vi "gascell.vi"() -> ()   [LabVIEW 2014, in "Panels.lvlib"]
uses:
  Panels.lvlib
  CSlibraries-extern/DimLVEvent/DimIndicators/DimIndicators.lvlib
  CSlibraries/UtilityLib/UtilityLib.lvlib
  CSCore/CSSystem/CoreLib/CoreLib.lvlib
  CSlibraries/UtilityLib/UtilityLib.valueStatus.ctl
  CSlibraries-extern/DimLVEvent/LVDimInterface/LVDimInterface.lvlib
  Instance           1 15Saved   gascell .vi
  CSCore/CSSystem/CoreLib/CoreLib.string 2 byte array.vi
  CSCore/CSSystem/CoreLib/CoreLib.double 2 byte array.vi
  CSCore/CSSystem/CoreLib/CoreLib.short 2 byte array.vi
  CSlibraries-extern/DimLVEvent/DimIndicators/DimIndicators.numericType.ctl
  CSCore/BaseProcess/BaseProcess.descriptor string definition.ctl
  CSCore/BaseProcess/BaseProcess.lvlib
  CSCore/CSSystem/CoreDefs/CoreDefs.rawDataType.ctl
  CSCore/CSSystem/CoreDefs/CoreDefs.call_type.ctl
  CSlibraries-extern/DimLVEvent/DimIndicators/DimIndicators.numericArrayType.ctl
  CSlibraries-extern/DimLVEvent/DimIndicators/DimIndicators.anyType.ctl
panel:
  in  "ListOfBases_Data":T1={"data"="NOLINK", "no link"=TRUE, "quality"=-1, "timeStamp"=0.0}
  in  "SetFileLocation_Data":T1={"data"="NOLINK", "no link"=TRUE, "quality"=-1, "timeStamp"=0.0}
  in  "GasCellBase_SetValueInfoData":T2={"data"=[0.0, 400.0, 2.0], "no link"=FALSE, "quality"=0, "timeStamp"=3265902002.226}
  in  "Flower2":bool
  in  "Flower3":bool
  in  "NozzlePlate":bool
  in  "NozzleVolt":bool
  in  "Flower1":bool
  in  "Flower4":bool
  in  "Ring21":bool
  in  "Ring18":bool
  in  "Ring17":bool
  in  "Ring3":bool
  in  "Ring1":bool
  in  "GasCellPIR_MonData":T3={"data"=inf, "no link"=FALSE, "quality"=1, "timeStamp"=3265902002.211}
  in  "N4PumpPIR_MonData":T3={"data"=inf, "no link"=FALSE, "quality"=1, "timeStamp"=3265902002.211}
  out "GasCellPIR_Mon":dbl=inf format="%.4f"
  out "N4PumpPIR_Mon":dbl=inf format="%.4f"
  in  "NozzlePlate_SetValueInfoData":T2={"data"=[0.0, 400.0, 2.0], "no link"=FALSE, "quality"=0, "timeStamp"=3265902002.226}
  in  "GasCellBase_SetData":T2={"data"=[0.0, 0.0, 0.0, 0.0], "no link"=FALSE, "quality"=0, "timeStamp"=3265902003.554}
  in  "NozzleVolt_SetValueInfoData":T2={"data"=[-120.0, 120.0, 2.0], "no link"=FALSE, "quality"=0, "timeStamp"=3265902002.226}
  in  "NozzlePlate_SetData":T2={"data"=[0.0, 0.0, 0.0, 0.0], "no link"=FALSE, "quality"=0, "timeStamp"=3265902003.57}
  in  "NozzlePlate_MonData":T3={"data"=inf, "no link"=FALSE, "quality"=1, "timeStamp"=3265902002.195}
  out "Ring3_Mon":dbl=inf format="%.4f"
  out "Ring1_Mon":dbl=inf format="%.4f"
  out "i ref out":refnum<vi>
  in  "Last Loaded File_Data":T1
  out "FileUpToDate":bool=TRUE caption="Parameter Changed"
  in  "Close All Panels":bool
  in  "Ring3_SetValueInfoData":T2={"data"=[0.0, 2989.8, 2.0], "no link"=FALSE, "quality"=0, "timeStamp"=3265902002.211}
  in  "Ring17_SetValueInfoData":T2={"data"=[0.0, 2988.4, 2.0], "no link"=FALSE, "quality"=0, "timeStamp"=3265902002.226}
  in  "Ring18_SetValueInfoData":T2={"data"=[0.0, 2984.0, 2.0], "no link"=FALSE, "quality"=0, "timeStamp"=3265902002.226}
  in  "Ring21_SetValueInfoData":T2={"data"=[0.0, 1488.3, 2.0], "no link"=FALSE, "quality"=0, "timeStamp"=3265902002.226}
  in  "Flower1_SetValueInfoData":T2={"data"=[0.0, 1487.9, 2.0], "no link"=FALSE, "quality"=0, "timeStamp"=3265902002.226}
  in  "Flower2_SetValueInfoData":T2={"data"=[0.0, 1486.0, 2.0], "no link"=FALSE, "quality"=0, "timeStamp"=3265902002.226}
  in  "Flower3_SetValueInfoData":T2={"data"=[0.0, 1488.7, 2.0], "no link"=FALSE, "quality"=0, "timeStamp"=3265902002.226}
  in  "Flower4_SetValueInfoData":T2={"data"=[0.0, 500.0, -1.0], "no link"=FALSE, "quality"=0, "timeStamp"=3265902002.226}
  in  "Ring1_SetValueInfoData":T2={"data"=[0.0, 2997.3, 2.0], "no link"=FALSE, "quality"=0, "timeStamp"=3265902002.211}
  in  "Ring1_SetData":T2={"data"=[0.0, 0.0, 0.0, 0.0], "no link"=FALSE, "quality"=0, "timeStamp"=3265902003.554}
  in  "Flower4_SetData":T2={"data"=[0.0, 0.0, 0.0, 0.0], "no link"=FALSE, "quality"=0, "timeStamp"=3265902003.539}
  in  "Flower3_SetData":T2={"data"=[0.0, 0.0, 0.0, 0.0], "no link"=FALSE, "quality"=0, "timeStamp"=3265902003.57}
  in  "Flower2_SetData":T2={"data"=[0.0, 0.0, 0.0, 0.0], "no link"=FALSE, "quality"=0, "timeStamp"=3265902003.554}
  in  "Flower1_SetData":T2={"data"=[0.0, 0.0, 0.0, 0.0], "no link"=FALSE, "quality"=0, "timeStamp"=3265902003.554}
  in  "Ring21_SetData":T2={"data"=[0.0, 0.0, 0.0, 0.0], "no link"=FALSE, "quality"=0, "timeStamp"=3265902003.554}
  in  "Ring18_SetData":T2={"data"=[0.0, 0.0, 0.0, 0.0], "no link"=FALSE, "quality"=0, "timeStamp"=3265902003.554}
  in  "Ring17_SetData":T2={"data"=[0.0, 0.0, 0.0, 0.0], "no link"=FALSE, "quality"=0, "timeStamp"=3265902003.554}
  in  "Ring3_SetData":T2={"data"=[0.0, 0.0, 0.0, 0.0], "no link"=FALSE, "quality"=0, "timeStamp"=3265902003.554}
  in  "NozzleVolt_SetData":T2={"data"=[0.0, 0.0, 0.0, 0.0], "no link"=FALSE, "quality"=0, "timeStamp"=3265902003.57}
  in  "call cluster in":T4={"Object"="", "Selector"="", "CallType"=enum."synchronous", "Async Object"="", "Async Selector"="", "Data Descriptor"="", "Data"=[], "Error #"=0, "Expire"=0}
  in  "GasCellBase":dbl
  out "Last Loaded File":string
  in  "SetFileLocation":path=path "\\\\intranet\\Files/projects/lebit/Data Exchange/data/GasCellControl"
  in  "NozzleVolt_MonData":T3={"data"=inf, "no link"=FALSE, "quality"=1, "timeStamp"=3265902002.195}
  in  "Flower4_MonData":T3={"data"=inf, "no link"=FALSE, "quality"=1, "timeStamp"=3265902002.195}
  in  "Flower3_MonData":T3={"data"=inf, "no link"=FALSE, "quality"=1, "timeStamp"=3265902002.195}
  in  "Flower2_MonData":T3={"data"=inf, "no link"=FALSE, "quality"=1, "timeStamp"=3265902002.195}
  in  "Flower1_MonData":T3={"data"=inf, "no link"=FALSE, "quality"=1, "timeStamp"=3265902002.195}
  in  "Ring21_MonData":T3={"data"=inf, "no link"=FALSE, "quality"=1, "timeStamp"=3265902002.195}
  in  "Ring18_MonData":T3={"data"=inf, "no link"=FALSE, "quality"=1, "timeStamp"=3265902002.195}
  in  "Ring17_MonData":T3={"data"=inf, "no link"=FALSE, "quality"=1, "timeStamp"=3265902002.195}
  in  "Ring3_MonData":T3={"data"=inf, "no link"=FALSE, "quality"=1, "timeStamp"=3265902002.195}
  in  "Ring1_MonData":T3={"data"=inf, "no link"=FALSE, "quality"=1, "timeStamp"=3265902002.195}
  out "NozzlePlate_Mon":dbl=inf format="%.4f"
  out "Flower1_Mon":dbl=inf format="%.4f"
  out "Ring17_Mon":dbl=inf format="%.4f"
  out "Flower2_Mon":dbl=inf format="%.4f"
  out "Ring21_Mon":dbl=inf format="%.4f"
  out "Flower4_Mon":dbl=inf format="%.4f"
  out "Ring18_Mon":dbl=inf format="%.4f"
  out "NozzleVolt_Mon":dbl=inf format="%.4f"
  out "Flower3_Mon":dbl=inf format="%.4f"
  # "Parameter changed, data file is no longer up-to-date."
  # "GasCellPIR"
  # "N4PumpPIR"
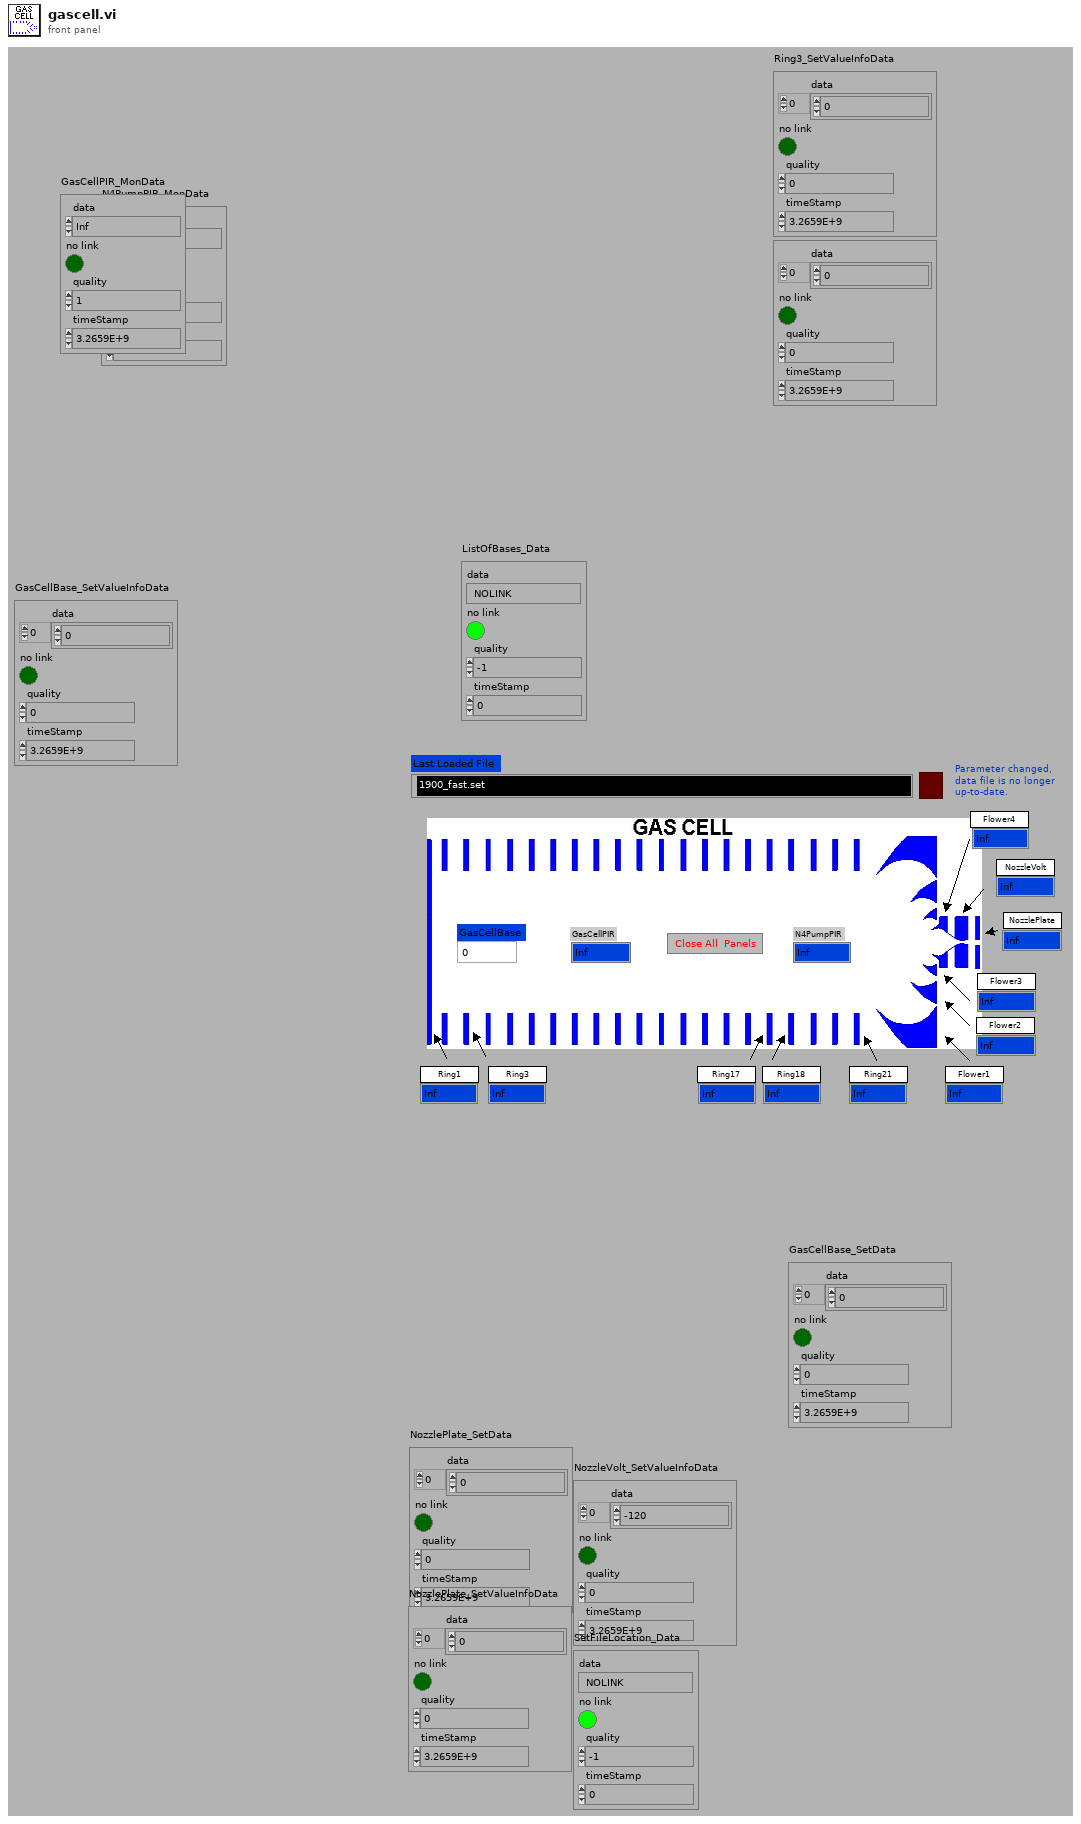
[diagram p1: front panel]
types:
  T1 = typedef "DimIndicators.lvlib/DimIndicators.anyType.ctl" = cluster{"data":string, "no link":bool, "quality":i32, "timeStamp":dbl}
  T2 = typedef "DimIndicators.lvlib/DimIndicators.numericArrayType.ctl" = cluster{"data":dbl[], "no link":bool, "quality":i32, "timeStamp":dbl}
  T3 = typedef "DimIndicators.lvlib/DimIndicators.numericType.ctl" = cluster{"data":dbl, "no link":bool, "quality":i32, "timeStamp":dbl}
  T4 = typedef "CoreDefs.call_type.ctl" = cluster{"Object":string, "Selector":string, "CallType":enum16{"simple", "synchronous", "asynchronous"}, "Async Object":string, "Async Selector":string, "Data Descriptor":T5, "Data":T6, "Error #":i32, "Expire":u32}
  T5 = typedef "BaseProcess.lvlib/BaseProcess.descriptor string definition.ctl" = string
  T6 = typedef "CoreDefs.rawDataType.ctl" = i8[]
  T7 = typedef "UtilityLib.lvlib/UtilityLib.valueStatus.ctl" = enum16{"no info available", "stand by/off", "on", "warning", "alarm/malfunction", "not implemented", "user action required", "important information", "system default", "control default", "indicator default", "button default"}
  T8 = cluster{"data":string, "no link":bool, "quality":i32, "timeStamp":dbl}
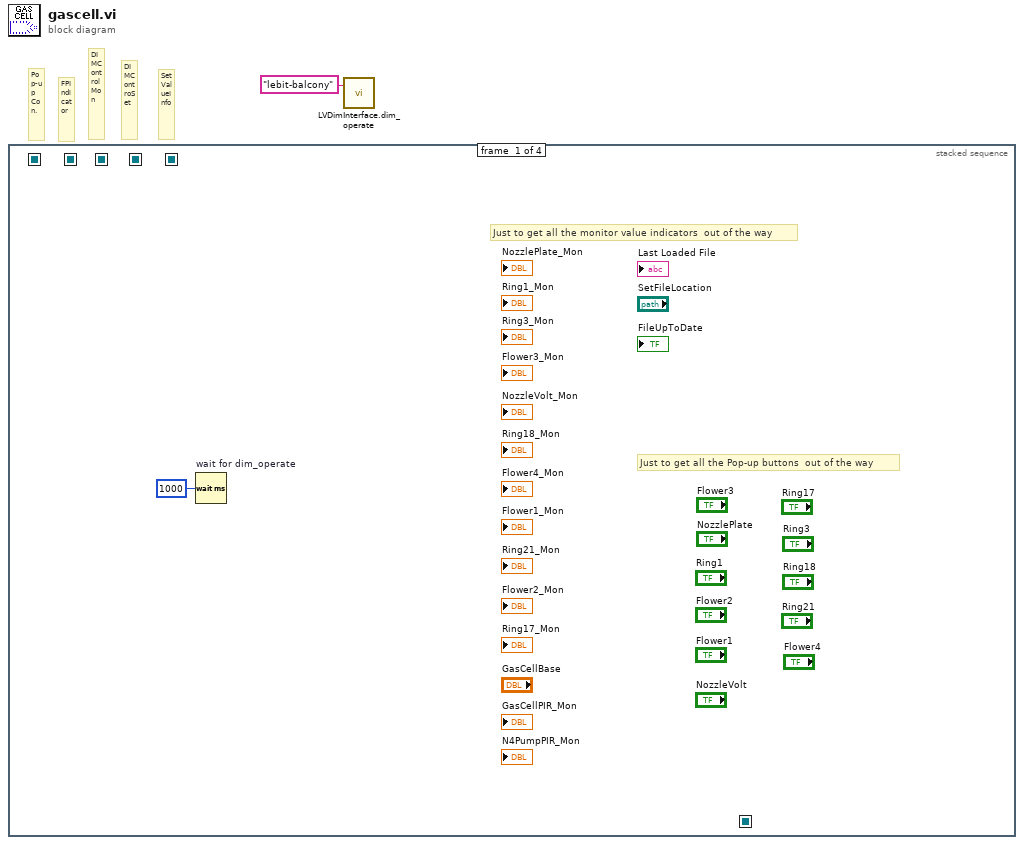
[diagram p0: block diagram]
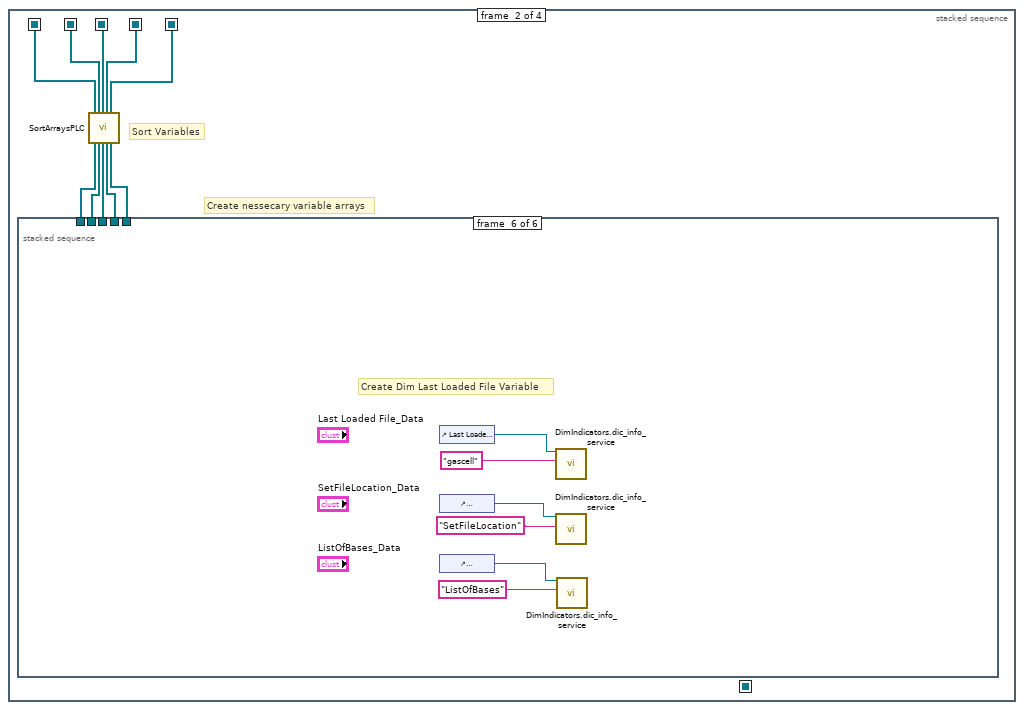
[diagram p2: hidden frame]
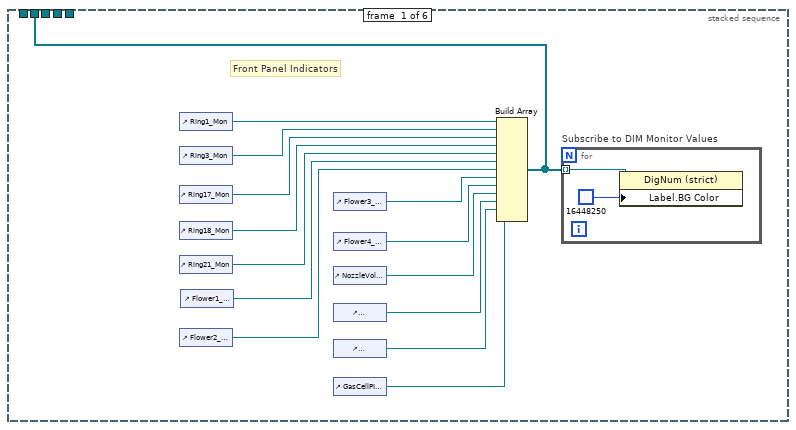
[diagram p3: hidden frame]
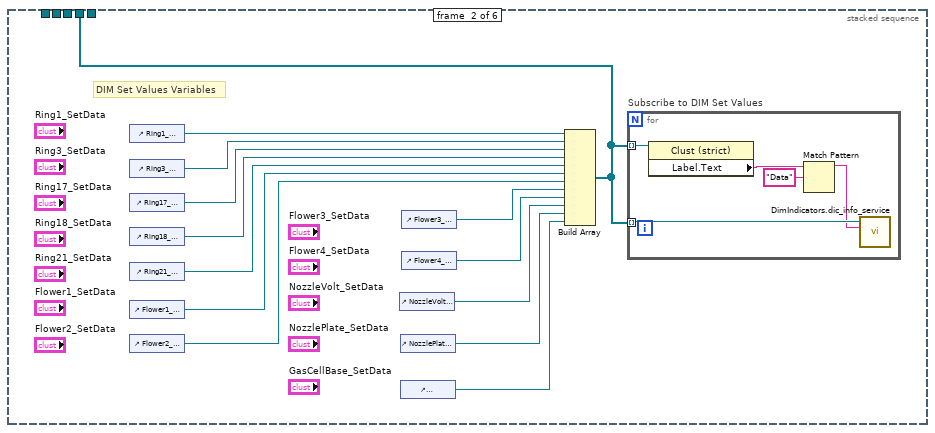
[diagram p4: hidden frame]
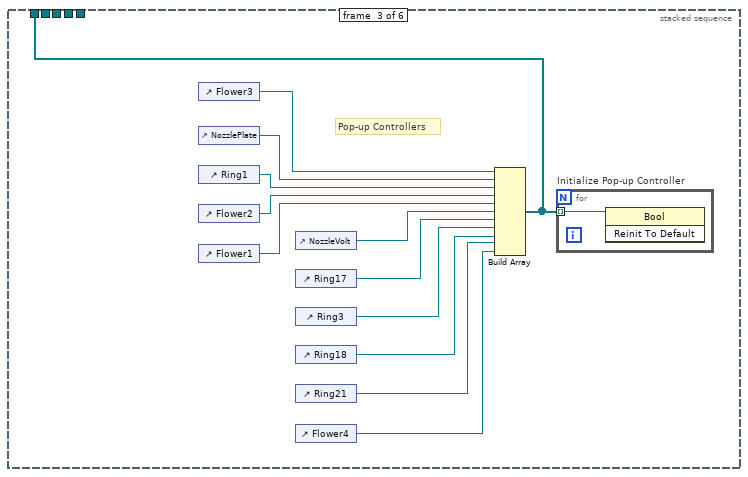
[diagram p5: hidden frame]
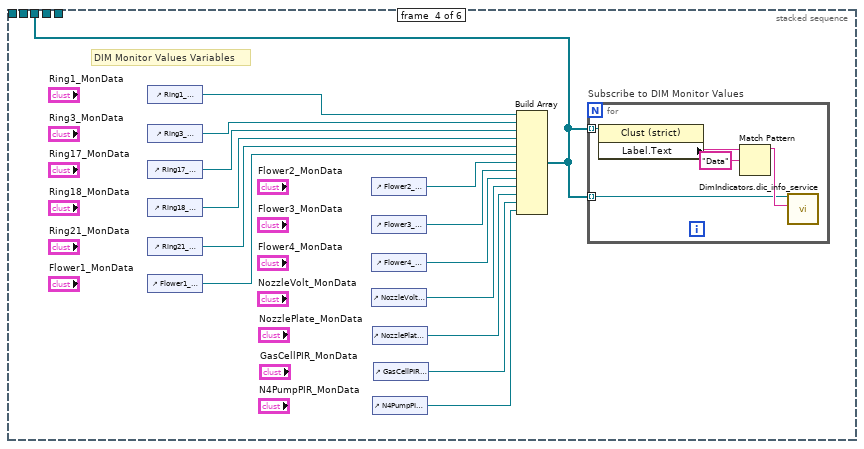
[diagram p6: hidden frame]
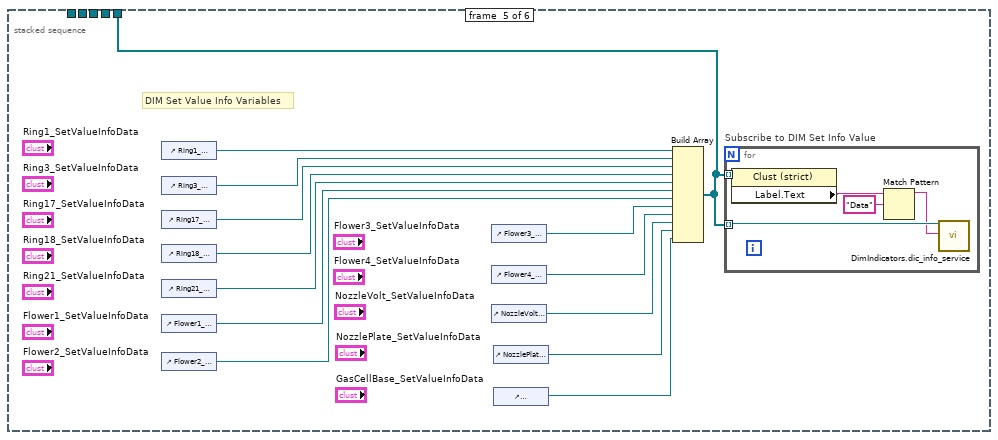
[diagram p7: hidden frame]
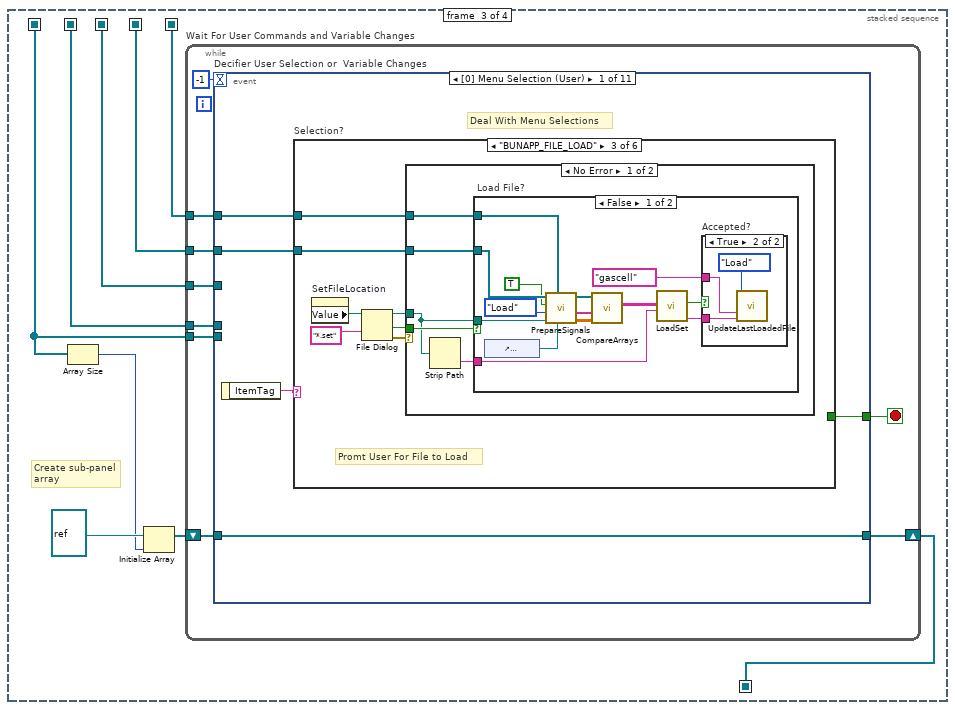
[diagram p8: hidden frame]
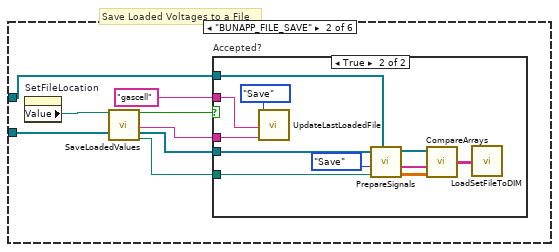
[diagram p10: hidden frame]
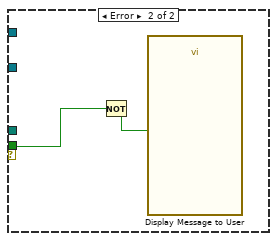
[diagram p14: hidden frame]
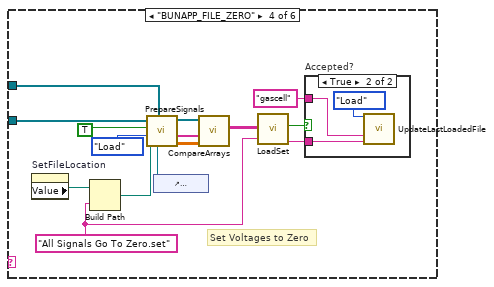
[diagram p15: hidden frame]
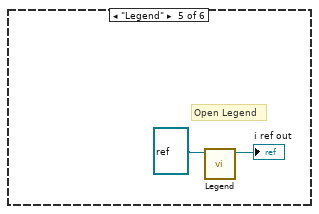
[diagram p17: hidden frame]
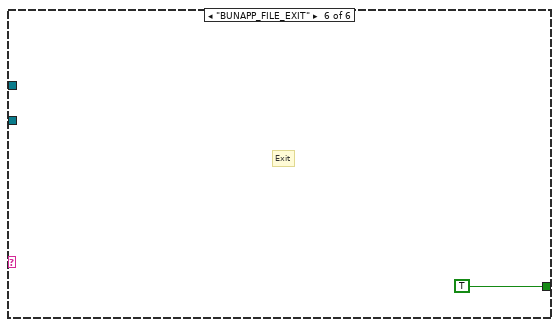
[diagram p18: hidden frame]
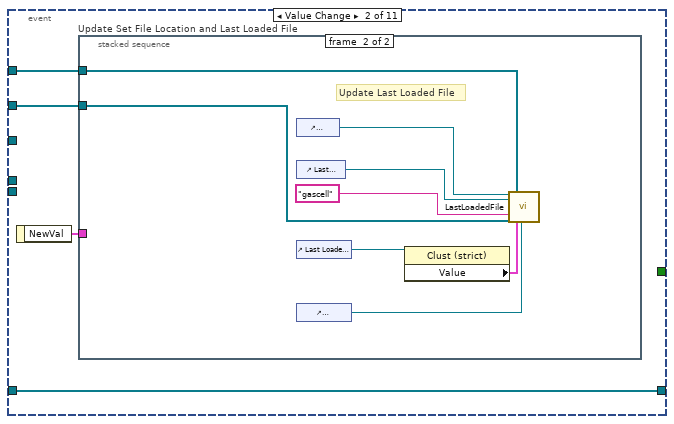
[diagram p19: hidden frame]
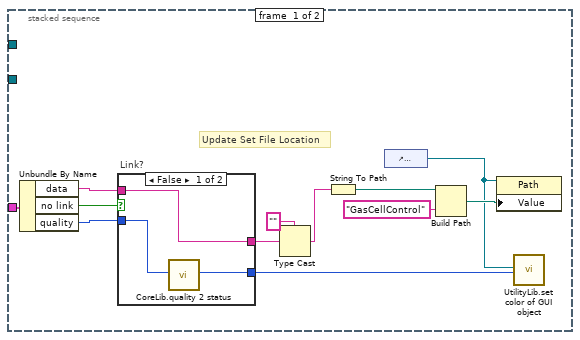
[diagram p20: hidden frame]
diagram:
  # "Pop-up Con."
  # "SetValueInfo"
  # "DIMControSet"
  # "DIMControlMon"
  # "FPIndicator"
  n1 = stacked-sequence {
    seq-local: [_ w11 _ _] -> [_ _ w108 _]
    seq-local: [_ w10 _ _] -> [_ _ w111 w352]
    seq-local: [_ _ w106 _] -> [_ _ _ w351]
    seq-local: [_ w9 _ _] -> [_ _ w105 w350]
    seq-local: [_ w8 _ _] -> [_ _ w104 w349]
    seq-local: [_ w12 _ _] -> [_ _ w103 _]
    frame #0 {
      # "Just to get all the Pop-up buttons  out of the way"
      # "Just to get all the monitor value indicators  out of the way"
      n2 = Wait (ms) "wait for dim_operate"(milliseconds to wait=u32 1000) -> ()  [unwired: 1 out]
    }
    frame #1 {
      # "Create nessecary variable arrays"
      # "Sort Variables"
      n3 = stacked-sequence {
        tunnel: [w13 _ _ _ _ _] -> w7
        tunnel: [_ w29 _ _ _ _] -> w6
        tunnel: [_ _ w47 _ _ _] -> w5
        tunnel: [_ _ _ w60 _ _] -> w4
        tunnel: [_ _ _ _ w79 _] -> w3
        frame #0 {
          # "Front Panel Indicators"
          n4 = control-ref of="Ring1_Mon"() -> (w26:refnum<vi>)
          n5 = control-ref of="Ring3_Mon"() -> (w24:refnum<vi>)
          n6 = control-ref of="Ring17_Mon"() -> (w21:refnum<vi>)
          n7 = control-ref of="Ring18_Mon"() -> (w20:refnum<vi>)
          n8 = control-ref of="Ring21_Mon"() -> (w14:refnum<vi>)
          n9 = control-ref of="Flower2_Mon"() -> (w16:refnum<vi>)
          n10 = control-ref of="Flower1_Mon"() -> (w15:refnum<vi>)
          n11 = control-ref of="Flower3_Mon"() -> (w17:refnum<vi>)
          n12 = control-ref of="Flower4_Mon"() -> (w18:refnum<vi>)
          n13 = control-ref of="NozzleVolt_Mon"() -> (w19:refnum<vi>)
          n14 = control-ref of="NozzlePlate_Mon"() -> (w25:refnum<vi>)
          n15 = control-ref of="N4PumpPIR_Mon"() -> (w23:refnum<vi>)
          n16 = control-ref of="GasCellPIR_Mon"() -> (w22:refnum<vi>)
          n17 = Build Array(w26, w24, w21, w20, w14, w15, w16, w17, w18, w19, w25, w23, w22) -> (w13:refnum<vi>[])
          n18 = for "Subscribe to DIM Monitor Values" {
            tunnel: w13 -> [w28] mode=indexing
            n19 = property class="DigNum (strict)"(reference=w28, "Label.BG Color"=u32 16448250 ("Color Box")) -> ()  [unwired: 1 in, 2 out]
          }
        }
        frame #1 {
          # "DIM Set Values Variables"
          n20 = control-ref of="Ring1_SetData"() -> (w41:refnum<vi>)
          n21 = control-ref of="Ring3_SetData"() -> (w40:refnum<vi>)
          n22 = control-ref of="Ring17_SetData"() -> (w39:refnum<vi>)
          n23 = control-ref of="Ring18_SetData"() -> (w38:refnum<vi>)
          n24 = control-ref of="Ring21_SetData"() -> (w37:refnum<vi>)
          n25 = control-ref of="Flower1_SetData"() -> (w36:refnum<vi>)
          n26 = control-ref of="Flower2_SetData"() -> (w35:refnum<vi>)
          n27 = control-ref of="NozzleVolt_SetData"() -> (w32:refnum<vi>)
          n28 = control-ref of="NozzlePlate_SetData"() -> (w31:refnum<vi>)
          n29 = control-ref of="GasCellBase_SetData"() -> (w30:refnum<vi>)
          n30 = control-ref of="Flower3_SetData"() -> (w34:refnum<vi>)
          n31 = control-ref of="Flower4_SetData"() -> (w33:refnum<vi>)
          n32 = Build Array(w41, w40, w39, w38, w37, w36, w35, w34, w33, w32, w31, w30) -> (w29:refnum<vi>[])
          n33 = for "Subscribe to DIM Set Values" {
            tunnel: w29 -> [w42] mode=indexing
            tunnel: w29 -> [w46] mode=indexing
            n34 = property class="Clust (strict)"(reference=w42) -> ("Label.Text"=w45:string)  [unwired: 1 in, 2 out]
            n35 = Match Pattern(string=w45, regular expression="Data") -> (before substring=w43:string)  [unwired: 1 in, 3 out]
            n36 = call "DimIndicators.dic_info_service.vi"("controlRef"=w46, "serviceName"=w43) -> ()  [unwired: 16 in, 2 out]
          }
        }
        frame #2 {
          # "Pop-up Controllers"
          n37 = control-ref of="Flower3"() -> (w58:refnum<vi>)
          n38 = control-ref of="NozzlePlate"() -> (w57:refnum<vi>)
          n39 = control-ref of="Ring1"() -> (w56:refnum<vi>)
          n40 = control-ref of="Flower2"() -> (w55:refnum<vi>)
          n41 = control-ref of="Flower1"() -> (w54:refnum<vi>)
          n42 = control-ref of="NozzleVolt"() -> (w53:refnum<vi>)
          n43 = control-ref of="Ring17"() -> (w52:refnum<vi>)
          n44 = control-ref of="Ring3"() -> (w51:refnum<vi>)
          n45 = control-ref of="Ring18"() -> (w50:refnum<vi>)
          n46 = control-ref of="Ring21"() -> (w49:refnum<vi>)
          n47 = control-ref of="Flower4"() -> (w48:refnum<vi>)
          n48 = Build Array(w58, w57, w56, w55, w54, w53, w52, w51, w50, w49, w48) -> (w47:refnum<vi>[])
          n49 = for "Initialize Pop-up Controller" {
            tunnel: w47 -> [w59] mode=indexing
            n50 = invoke class="Bool" method="Reinit To Default"(reference=w59) -> ()  [unwired: 2 in, 3 out]
          }
        }
        frame #3 {
          # "DIM Monitor Values Variables"
          n51 = control-ref of="Ring1_MonData"() -> (w73:refnum<vi>)
          n52 = control-ref of="Ring3_MonData"() -> (w72:refnum<vi>)
          n53 = control-ref of="Ring17_MonData"() -> (w71:refnum<vi>)
          n54 = control-ref of="Ring18_MonData"() -> (w70:refnum<vi>)
          n55 = control-ref of="Ring21_MonData"() -> (w69:refnum<vi>)
          n56 = control-ref of="Flower1_MonData"() -> (w68:refnum<vi>)
          n57 = control-ref of="Flower2_MonData"() -> (w67:refnum<vi>)
          n58 = control-ref of="Flower3_MonData"() -> (w66:refnum<vi>)
          n59 = control-ref of="Flower4_MonData"() -> (w61:refnum<vi>)
          n60 = control-ref of="NozzleVolt_MonData"() -> (w63:refnum<vi>)
          n61 = control-ref of="NozzlePlate_MonData"() -> (w62:refnum<vi>)
          n62 = control-ref of="N4PumpPIR_MonData"() -> (w64:refnum<vi>)
          n63 = control-ref of="GasCellPIR_MonData"() -> (w65:refnum<vi>)
          n64 = Build Array(w73, w72, w71, w70, w69, w68, w67, w66, w61, w63, w62, w65, w64) -> (w60:refnum<vi>[])
          n65 = for "Subscribe to DIM Monitor Values" {
            tunnel: w60 -> [w75] mode=indexing
            tunnel: w60 -> [w74] mode=indexing
            n66 = property class="Clust (strict)"(reference=w74) -> ("Label.Text"=w77:string)  [unwired: 1 in, 2 out]
            n67 = Match Pattern(string=w77, regular expression="Data") -> (before substring=w76:string)  [unwired: 1 in, 3 out]
            n68 = call "DimIndicators.dic_info_service.vi"("controlRef"=w75, "serviceName"=w76) -> ()  [unwired: 16 in, 2 out]
          }
        }
        frame #4 {
          # "DIM Set Value Info Variables"
          n69 = control-ref of="Ring1_SetValueInfoData"() -> (w91:refnum<vi>)
          n70 = control-ref of="Ring3_SetValueInfoData"() -> (w90:refnum<vi>)
          n71 = control-ref of="Ring17_SetValueInfoData"() -> (w89:refnum<vi>)
          n72 = control-ref of="Ring18_SetValueInfoData"() -> (w88:refnum<vi>)
          n73 = control-ref of="Ring21_SetValueInfoData"() -> (w87:refnum<vi>)
          n74 = control-ref of="Flower1_SetValueInfoData"() -> (w86:refnum<vi>)
          n75 = control-ref of="Flower2_SetValueInfoData"() -> (w85:refnum<vi>)
          n76 = control-ref of="Flower3_SetValueInfoData"() -> (w84:refnum<vi>)
          n77 = control-ref of="Flower4_SetValueInfoData"() -> (w83:refnum<vi>)
          n78 = control-ref of="NozzleVolt_SetValueInfoData"() -> (w82:refnum<vi>)
          n79 = control-ref of="NozzlePlate_SetValueInfoData"() -> (w81:refnum<vi>)
          n80 = control-ref of="GasCellBase_SetValueInfoData"() -> (w80:refnum<vi>)
          n81 = Build Array(w91, w90, w89, w88, w87, w86, w85, w84, w83, w82, w81, w80) -> (w79:refnum<vi>[])
          n82 = for "Subscribe to DIM Set Info Value" {
            tunnel: w79 -> [w92] mode=indexing
            tunnel: w79 -> [w96] mode=indexing
            n83 = property class="Clust (strict)"(reference=w92) -> ("Label.Text"=w95:string)  [unwired: 1 in, 2 out]
            n84 = Match Pattern(string=w95, regular expression="Data") -> (before substring=w93:string)  [unwired: 1 in, 3 out]
            n85 = call "DimIndicators.dic_info_service.vi"("controlRef"=w96, "serviceName"=w93) -> ()  [unwired: 16 in, 2 out]
          }
        }
        frame #5 {
          # "Create Dim Last Loaded File Variable"
          n86 = control-ref of="Last Loaded File_Data"() -> (w100:refnum<vi>)
          n87 = control-ref of="SetFileLocation_Data"() -> (w102:refnum<vi>)
          n88 = control-ref of="ListOfBases_Data"() -> (w98:refnum<vi>)
          n89 = call "DimIndicators.dic_info_service.vi"("controlRef"=w100, "serviceName"="gascell" ("string")) -> ()  [unwired: 16 in, 2 out]
          n90 = call "DimIndicators.dic_info_service.vi"("controlRef"=w102, "serviceName"="SetFileLocation" ("string")) -> ()  [unwired: 16 in, 2 out]
          n91 = call "DimIndicators.dic_info_service.vi"("controlRef"=w98, "serviceName"="ListOfBases" ("string")) -> ()  [unwired: 16 in, 2 out]
        }
      }
      n92 = call "SortArraysPLC.vi"("Pop-up Con."=w5, "FPIndicator in"=w7, "DIMControlMon"=w4, "DIMControSet"=w6, "SetValueInfo"=w3) -> ("Pop-up Con. out"=w12:refnum<vi>[], "FPIndicator out"=w11:refnum<vi>[], "DIMControlMon out"=w10:refnum<vi>[], "DIMControSet out"=w9:refnum<vi>[], "SetValueInfo out"=w8:refnum<vi>[])  [unwired: 18 in]
    }
    frame #2 {
      # "Create sub-panel\narray"
      n93 = Array Size(array=w103) -> (size(s)=w107:i32)
      n94 = Initialize Array(refnum<vi> refnum ("vi reference"), w107) -> (w110:refnum<vi>[])
      n95 = while "Wait For User Commands and Variable Changes" {
        tunnel: w111 -> [w119]
        tunnel: w108 -> [w118]
        shift-right: [w116] -> w106
        shift-left: w110 -> [w117]
        tunnel: w105 -> [w115]
        tunnel: w104 -> [w114]
        tunnel: w103 -> [w112]
        stop <- w120 stop-if-true
        n96 = event "Decifier User Selection or  Variable Changes" shown="[0] Menu Selection (User)" {
          selector: _ -> [_ _ _ _ _ _ _ _ _ _ _]
          dyn-events: _ -> [_ _ _ _ _ _ _ _ _ _ _]
          timeout: -1 -> [_ _ _ _ _ _ _ _ _ _ _]
          tunnel: [w122 _ _ _ _ _ _ _ _ _ TRUE ("stop")] -> w120
          tunnel: w119 -> [_ _ _ _ _ w281 _ _ _ _ w324]
          tunnel: w118 -> [_ _ _ _ _ w279 _ _ _ _ _]
          tunnel: w117 -> [w125 w198 w233 w240 w263 w283 w301 w309 w316 w322 w323]
          tunnel: [w125 w198 w233 w240 w263 w283 w301 w307 w314 w322 _] -> w116
          tunnel: w115 -> [w123 w199 w231 w241 w260 _ w300 _ _ _ w325]
          tunnel: w114 -> [w121 w197 w227 w242 _ _ _ _ _ _ w326]
          tunnel: w112 -> [_ _ _ _ _ _ _ w303 _ _ _]
          event Menu Selection (User) {
            # "Deal With Menu Selections"
            n97 = event-data() -> ("ItemTag"=w124:string)  [unwired: 1 in]
            n98 = case "Selection?" shown="\"BUNAPP_FILE_LOAD\"" w124 {
              tunnel: w123 -> [_ w130 w150 w190 _ _]
              tunnel: [_ _ _ _ _ TRUE ("stop")] -> w122
              tunnel: w121 -> [_ w126 w145 w177 _ _]
              frame "False", Default {
              }
              frame "BUNAPP_FILE_SAVE" {
                # "Save Loaded Voltages to a File"
                n99 = property on="SetFileLocation" class="Path"() -> ("Value"=w131:path)  [unwired: 2 in, 2 out]
                n100 = call "SaveLoadedValues.vi"("Panel Location?"=w131, "DIMControlSet in"=w130) -> ("File Saved?"=w132:bool, "File Name"=w129:string, "DIMControlSet out"=w127:refnum<vi>[], "Path"=w128:path)  [unwired: 14 in]
                n101 = case "Accepted?" shown="True" w132 {
                  tunnel: w129 -> [_ w142]
                  tunnel: "gascell" ("string") -> [_ w144]
                  tunnel: w127 -> [_ w143]
                  tunnel: w128 -> [_ w141]
                  tunnel: w126 -> [_ w135]
                  frame False {
                  }
                  frame True {
                    n102 = call "UpdateLastLoadedFile.vi"("LoadOrSave"=enum16{"Load", "Save"}."Save", "GUIName"=w144, "FileNameIn"=w142) -> ()  [unwired: 13 in]
                    n103 = call "PrepareSignals.vi"("SetValueInfo in"=w135, "setfile path"=w141, "Enum"=enum16{"Save", "Load"}."Save", "DIMControSet in"=w143) -> ("indexed loaded Array"=w139:dbl[][], "Name Array"=w140:string[], "DIMControSet out"=w138:refnum<vi>[])  [unwired: 5 in]
                    n104 = call "CompareArrays.vi"("indexed loaded Array"=w139, "Name Array"=w140, "DIMControSet"=w138) -> ("Table for loading values"=w137:string[][])  [unwired: 4 in]
                    n105 = call "LoadSetFileToDIM.vi"("output array"=w137) -> ()  [unwired: 2 in]
                  }
                }
              }
              frame "BUNAPP_FILE_LOAD" {
                # "Promt User For File to Load"
                n106 = property on="SetFileLocation" class="Path"() -> ("Value"=w147:path)  [unwired: 2 in, 2 out]
                n107 = File Dialog(6:"*.set" ("pattern (all files)"), 11:w147) -> (0:w146:errorcluster, 1:w151:bool, 3:w148:path)  [unwired: 5 in, 1 out]
                n108 = case shown="No Error" w146 {
                  tunnel: w151 -> [w156 w174]
                  tunnel: w150 -> [w155 _]
                  tunnel: w148 -> [w153 _]
                  tunnel: w145 -> [w152 _]
                  frame No Error {
                    n109 = Strip Path(path=w153) -> (name=w154:string)  [unwired: 1 out]
                    n110 = case "Load File?" shown="False" w156 {
                      tunnel: w155 -> [w170 _]
                      tunnel: w154 -> [w164 _]
                      tunnel: w153 -> [w165 _]
                      tunnel: w152 -> [w158 _]
                      frame False {
                        n111 = control-ref of="ListOfBases_Data"() -> (w157:refnum<vi>)
                        n112 = call "PrepareSignals.vi"("ListOfBases_Data"=w157, "SetValueInfo in"=w158, "setfile path"=w165, "Enum"=enum16{"Save", "Load"}."Load", "Display Message to \nUser"=TRUE ("Display Message to \nUser"), "DIMControSet in"=w170) -> ("indexed loaded Array"=w168:dbl[][], "Name Array"=w167:string[], "DIMControSet out"=w169:refnum<vi>[])  [unwired: 3 in]
                        n113 = call "CompareArrays.vi"("indexed loaded Array"=w168, "Name Array"=w167, "DIMControSet"=w169) -> ("Table for loading values"=w166:string[][])  [unwired: 4 in]
                        n114 = call "LoadSet.vi"("File Name In"=w164, "output array"=w166) -> ("File Name out"=w163:string, "Accepted"=w162:bool)  [unwired: 8 in]
                        n115 = case "Accepted?" shown="True" w162 {
                          tunnel: w163 -> [_ w173]
                          tunnel: "gascell" ("string") -> [_ w172]
                          frame False {
                          }
                          frame True {
                            n116 = call "UpdateLastLoadedFile.vi"("LoadOrSave"=enum16{"Load", "Save"}."Load", "GUIName"=w172, "FileNameIn"=w173) -> ()  [unwired: 13 in]
                          }
                        }
                      }
                      frame True {
                      }
                    }
                  }
                  frame Error {
                    n117 = Not(x=w174) -> (.not. x?=w175:bool)
                    n118 = call "Display Message to User"("Enable"=w175) -> ()  [unwired: 9 in, 2 out]
                  }
                }
              }
              frame "BUNAPP_FILE_ZERO" {
                w181 = "All Signals Go To Zero.set" ("File Name")
                # "Set Voltages to Zero"
                n119 = property on="SetFileLocation" class="Path"() -> ("Value"=w179:path)  [unwired: 2 in, 2 out]
                n120 = Build Path(base path=w179, name or relative path=w181) -> (appended path=w180:path)
                n121 = control-ref of="ListOfBases_Data"() -> (w176:refnum<vi>)
                n122 = call "PrepareSignals.vi"("ListOfBases_Data"=w176, "SetValueInfo in"=w177, "setfile path"=w180, "Enum"=enum16{"Save", "Load"}."Load", "Display Message to \nUser"=TRUE ("Display Message to \nUser"), "DIMControSet in"=w190) -> ("indexed loaded Array"=w188:dbl[][], "Name Array"=w187:string[], "DIMControSet out"=w189:refnum<vi>[])  [unwired: 3 in]
                n123 = call "CompareArrays.vi"("indexed loaded Array"=w188, "Name Array"=w187, "DIMControSet"=w189) -> ("Table for loading values"=w186:string[][])  [unwired: 4 in]
                n124 = call "LoadSet.vi"("File Name In"=w181, "output array"=w186) -> ("File Name out"=w184:string, "Accepted"=w185:bool)  [unwired: 8 in]
                n125 = case "Accepted?" shown="True" w185 {
                  tunnel: w184 -> [_ w193]
                  tunnel: "gascell" ("string") -> [_ w192]
                  frame False {
                  }
                  frame True {
                    n126 = call "UpdateLastLoadedFile.vi"("LoadOrSave"=enum16{"Load", "Save"}."Load", "GUIName"=w192, "FileNameIn"=w193) -> ()  [unwired: 13 in]
                  }
                }
              }
              frame "Legend" {
                # "Open Legend"
                n127 = call "Legend.vi"("i ref in"=refnum<vi> refnum) -> ("i ref out"=→"i ref out":refnum<vi>)  [unwired: 10 in]
              }
              frame "BUNAPP_FILE_EXIT" {
                # "Exit"
              }
            }
          }
          event Value Change {
            n128 = event-data() -> ("NewVal"=w200:T1)  [unwired: 1 in]
            n129 = stacked-sequence "Update Set File Location and Last Loaded File" {
              tunnel: w200 -> [w202 _]
              tunnel: w199 -> [_ w223]
              tunnel: w197 -> [_ w219]
              frame #0 {
                # "Update Set File Location"
                n130 = Unbundle By Name(w202) -> ("data"=w211:string, "no link"=w210:bool, "quality"=w209:i32)
                n131 = case "Link?" shown="False" w210 {
                  tunnel: w209 -> [w215 _]
                  tunnel: [w214 UtilityLib.valueStatus."no info available" ("valueStatus")] -> w212
                  tunnel: w211 -> [w213 _]
                  tunnel: [w213 w216] -> w207
                  frame False {
                    n132 = call "CoreLib.quality 2 status.vi"("quality"=w215) -> ("valueStatus"=w214:T7)  [unwired: 18 in]
                  }
                  frame True {
                    n133 = call "EmptyString.vi"() -> ("String"=w216:string)
                  }
                }
                n134 = Type Cast(type="" ("regular expression"), x=w207) -> (*(type *) &x=w206:string)
                n135 = String To Path(string=w206) -> (path=w203:path)
                n136 = control-ref of="SetFileLocation"() -> (w201:refnum<vi>)
                n137 = Build Path(base path=w203, name or relative path="GasCellControl") -> (appended path=w204:path)
                n138 = property class="Path"(reference=w201, "Value"=w204) -> ()  [unwired: 1 in, 2 out]
                n139 = call "UtilityLib.set color of GUI object.vi"("GUI object Ref"=w201, "valueStatus"=w212) -> ()  [unwired: 17 in, 1 out]
              }
              frame #1 {
                # "Update Last Loaded File"
                n140 = control-ref of="SetFileLocation"() -> (w222:refnum<vi>)
                n141 = control-ref of="Last Loaded File"() -> (w221:refnum<vi>)
                n142 = control-ref of="Last Loaded File_Data"() -> (w220:refnum<vi>)
                n143 = control-ref of="ListOfBases_Data"() -> (w218:refnum<vi>)
                n144 = property class="Clust (strict)"(reference=w220) -> ("Value"=w225:T8)  [unwired: 1 in, 2 out]
                n145 = call "LastLoadedFile.vi"("SetFileLocation"=w222, "Last Loaded File"=w221, "GUIName"="gascell", "DIMControSet in"=w223, "SetValueInfo in"=w219, "NewVal"=w225, "ListOfBases_Data"=w218) -> ()  [unwired: 13 in]
              }
            }
          }
          event Value Change {
            # "Update Last Loaded File"
            n146 = event-data() -> ("NewVal"=w232:T1)  [unwired: 1 in]
            n147 = control-ref of="Last Loaded File"() -> (w229:refnum<vi>)
            n148 = control-ref of="SetFileLocation"() -> (w230:refnum<vi>)
            n149 = control-ref of="ListOfBases_Data"() -> (w226:refnum<vi>)
            n150 = call "LastLoadedFile.vi"("SetFileLocation"=w230, "Last Loaded File"=w229, "GUIName"="gascell", "DIMControSet in"=w231, "SetValueInfo in"=w227, "NewVal"=w232, "ListOfBases_Data"=w226) -> ()  [unwired: 13 in]
          }
          event "GasCellBase": Value Change {
            w234 = "GasCellBase" ("string")
            # "Is Base in Range?"
            # "Update  Set Values"
            n151 = event-data() -> ("NewVal"=w237:dbl, "OldVal"=w236:dbl)  [unwired: 1 in, 4 out]
            n152 = control-ref of="ListOfBases_Data"() -> (w235:refnum<vi>)
            n153 = call "IsBaseInRange.vi"("SetValueInfo"=w242, "DIMControSet"=w241, "ListOfBases_Data"=w235, "NewVal in"=w237, "Base Name"=w234) -> ("NewVal Out"=w238:dbl, "In Range"=w239:bool)  [unwired: 13 in]
            n154 = case "Base In Range?" shown="True" w239 {
              tunnel: w238 -> [_ w245]
              tunnel: w236 -> [w243 _]
              tunnel: w234 -> [_ w244]
              frame False {
                n155 = property on="GasCellBase" class="DigNum (strict)"("Value"=w243) -> ()  [unwired: 2 in, 2 out]
              }
              frame True {
                n156 = call-poly "CoreLib.data 2 byte array.vi"("i16"=i16 0 ("element")) -> ("byteArray out"=w247:T6)  [unwired: 18 in]
                n157 = property on="GasCellBase" class="DigNum (strict)"("Value"=w245) -> ()  [unwired: 2 in, 2 out]
                n158 = call-poly "CoreLib.data 2 byte array.vi"("byteArray"=w247, "f64"=w245) -> ("byteArray out"=w251:T6)  [unwired: 17 in]
                n159 = Flatten To String(anything=TRUE) -> (data string=w250:string)  [unwired: 3 in, 2 out]
                n160 = Concatenate Strings("SetPLC" ("string"), w244) -> (w256:string)
                n161 = call-poly "CoreLib.data 2 byte array.vi"("byteArray"=w251, "string"=w250) -> ("byteArray out"=w248:T6)  [unwired: 17 in]
                n162 = Bundle By Name(cluster="call cluster in", "Object"="PLC", "Selector"=w256, "CallType"=enum16{"simple", "synchronous", "asynchronous"}."simple", "Data"=w248) -> (w253:T4)
                n163 = call "CoreLib.call process.vi"("call cluster in"=w253) -> ()  [unwired: 13 in, 2 out]
              }
            }
          }
          event Value Change {
            n164 = event-data() -> ("CtlRef"=w259:refnum<vi>, "NewVal"=w265:T2)  [unwired: 1 in, 4 out]
            n165 = Unbundle By Name(w265) -> ("data"=w266:dbl[], "no link"=w267:bool, "quality"=w269:i32)
            n166 = property on="FileUpToDate" class="Bool (strict)"() -> ("Value"=w258:bool)  [unwired: 2 in, 2 out]
            n167 = case "Link?" shown="True" w267 {
              tunnel: w269 -> [w271 _]
              tunnel: [w270 UtilityLib.valueStatus."no info available" ("valueStatus")] -> w268
              tunnel: w266 -> [w273 _]
              tunnel: [w272 inf] -> w262
              frame False {
                n168 = call "CoreLib.quality 2 status.vi"("quality"=w271) -> ("valueStatus"=w270:T7)  [unwired: 18 in]
                n169 = Index Array(array=w273, index #1=0 ("index")) -> (element #1=w272:dbl)  [unwired: 1 in, 1 out]
              }
              frame True {
              }
            }
            n170 = call "FileUpToDate.vi"("FileUpToDate in"=w258, "DIMControSet out"=w260, "CtlRef"=w259) -> ("FileUpToDate out"=w261:bool)  [unwired: 16 in]
            n171 = property on="FileUpToDate" class="Bool (strict)"("Value"=w261) -> ()  [unwired: 2 in, 2 out]
            n172 = control-ref of="GasCellBase"() -> (w264:refnum<vi>)
            n173 = property on="GasCellBase" class="DigNum (strict)"("Value"=w262) -> ()  [unwired: 2 in, 2 out]
            n174 = call "UtilityLib.set color of GUI object.vi"("GUI object Ref"=w264, "valueStatus"=w268) -> ()  [unwired: 17 in, 1 out]
          }
          event Value Change {
            # "Find Monitor Value Index"
            # "Updating a Monitor Value"
            n175 = event-data() -> ("CtlRef"=w280:refnum<vi>, "NewVal"=w284:T3)  [unwired: 1 in, 4 out]
            n176 = Search 1D Array(1D array=w281, element=w280) -> (index of element=w282:i32)  [unwired: 1 in]
            n177 = Index Array(array=w279, index=w282) -> (element=w277:refnum<vi>)
            n178 = Not A Number/Path/Refnum?(number/path/refnum=w277) -> (NaN/Path/Refnum?=w278:bool)
            n179 = case "Indicator does not exists?" shown="False" w278 {
              tunnel: w284 -> [_ w291]
              tunnel: w277 -> [_ w285]
              frame True {
              }
              frame False {
                n180 = Unbundle By Name(w291) -> ("data"=w287:dbl, "no link"=w288:bool, "quality"=w290:i32)
                n181 = case shown="True" w288 {
                  tunnel: w290 -> [w294 _]
                  tunnel: [w293 UtilityLib.valueStatus."no info available" ("valueStatus")] -> w289
                  tunnel: w287 -> [w292 _]
                  tunnel: [w292 inf] -> w286
                  frame False {
                    n182 = call "CoreLib.quality 2 status.vi"("quality"=w294) -> ("valueStatus"=w293:T7)  [unwired: 18 in]
                  }
                  frame True {
                  }
                }
                n183 = property class="DigNum (strict)"(reference=w285, "Value"=w286) -> ()  [unwired: 1 in, 2 out]
                n184 = call "TextColor.vi"("valueStatus"=w289, "reference"=w285) -> ()  [unwired: 10 in]
              }
            }
          }
          event Value Change {
            n185 = event-data() -> ("CtlRef"=w299:refnum<vi>)  [unwired: 1 in, 5 out]
            n186 = property on="FileUpToDate" class="Bool (strict)"() -> ("Value"=w297:bool)  [unwired: 2 in, 2 out]
            n187 = call "FileUpToDate.vi"("FileUpToDate in"=w297, "DIMControSet out"=w300, "CtlRef"=w299) -> ("FileUpToDate out"=w298:bool)  [unwired: 16 in]
            n188 = property on="FileUpToDate" class="Bool (strict)"("Value"=w298) -> ()  [unwired: 2 in, 2 out]
          }
          event "Ring1", "Ring3", "Ring17", "Ring18", "Ring21", "Flower4", "Flower1", "NozzleVolt", "NozzlePlate", "Flower3", "Flower2": Value Change {
            # "Find sub-panel index"
            # "opening or closing a sub-panel"
            n189 = event-data() -> ("CtlRef"=w302:refnum<vi>)  [unwired: 1 in, 3 out]
            n190 = Search 1D Array(1D array=w303, element=w302) -> (index of element=w308:i32)  [unwired: 1 in]
            n191 = Index Array(array=w309, index=w308) -> (element=w306:refnum<vi>)
            n192 = invoke class="Bool" method="Reinit To Default"(reference=w302) -> ()  [unwired: 2 in, 3 out]
            n193 = property class="VI"(reference=w306) -> ("Front Panel.Open"=w305:bool)  [unwired: 1 in, 2 out]
            n194 = case "Panel Already Open?" shown="False" w305 {
              tunnel: w302 -> [w310 _]
              tunnel: w306 -> [_ w313]
              tunnel: [w311 refnum<vi> refnum ("vi reference")] -> w304
              frame False {
                n195 = call "OpenPanel.vi"("CtlRef"=w310) -> ("vi reference"=w311:refnum<vi>)  [unwired: 2 in]
              }
              frame True {
                n196 = call "PanelClose.vi"("vi reference"=w313) -> ()
              }
            }
            n197 = Replace Array Subset(array=w309, new element=w304, index=w308) -> (w307:refnum<vi>[])
          }
          event "Close All Panels": Value Change {
            n198 = event-data() -> ()  [unwired: 1 in, 6 out]
            n199 = case "Close Open Panels?" shown="True" "Close All Panels" {
              tunnel: w316 -> [w317 w319]
              tunnel: [w317 w318] -> w314
              frame False {
              }
              frame True {
                n200 = for "Close Open Panels" {
                  tunnel: w319 -> [w321] mode=indexing
                  tunnel: w319 -> [w320]
                  tunnel: [w320] -> w318
                  n201 = call "PanelClose.vi"("vi reference"=w321) -> ()
                }
              }
            }
          }
          event Timeout {
            # "Timeout"
            n202 = event-data() -> ()  [unwired: 1 in, 3 out]
          }
          event Panel Close? {
            n203 = event-data() -> ()  [unwired: 1 in, 4 out]
            n204 = stacked-sequence {
              tunnel: w326 -> [w332 _]
              tunnel: w325 -> [w331 _]
              tunnel: w324 -> [w330 _]
              tunnel: w323 -> [w334 _]
              frame #0 {
                # "Release DIM Services"
                n205 = for "Close Open Panels" {
                  tunnel: w334 -> [w344] mode=indexing
                  n206 = call "PanelClose.vi"("vi reference"=w344) -> ()
                }
                n207 = for "For Each Service" {
                  tunnel: w331 -> [w339] mode=indexing
                  n208 = Not A Number/Path/Refnum?(number/path/refnum=w339) -> (NaN/Path/Refnum?=w338:bool)
                  n209 = case "Not a Reference?" shown="False" w338 {
                    tunnel: w339 -> [w340 _]
                    frame False {
                      n210 = call "DimIndicators.dic_release_service.vi"("controlRef"=w340) -> ()  [unwired: 18 in, 1 out]
                    }
                    frame True {
                    }
                  }
                }
                n211 = for "For Each Service" {
                  tunnel: w330 -> [w336] mode=indexing
                  n212 = Not A Number/Path/Refnum?(number/path/refnum=w336) -> (NaN/Path/Refnum?=w335:bool)
                  n213 = case "Not a Reference?" shown="False" w335 {
                    tunnel: w336 -> [w337 _]
                    frame False {
                      n214 = call "DimIndicators.dic_release_service.vi"("controlRef"=w337) -> ()  [unwired: 18 in, 1 out]
                    }
                    frame True {
                    }
                  }
                }
                n215 = for "For Each Service" {
                  tunnel: w332 -> [w342] mode=indexing
                  n216 = Not A Number/Path/Refnum?(number/path/refnum=w342) -> (NaN/Path/Refnum?=w341:bool)
                  n217 = case "Not a Reference?" shown="False" w341 {
                    tunnel: w342 -> [w343 _]
                    frame False {
                      n218 = call "DimIndicators.dic_release_service.vi"("controlRef"=w343) -> ()  [unwired: 18 in, 1 out]
                    }
                    frame True {
                    }
                  }
                }
                n219 = control-ref of="ListOfBases_Data"() -> (w328:refnum<vi>)
                n220 = control-ref of="SetFileLocation_Data"() -> (w329:refnum<vi>)
                n221 = control-ref of="Last Loaded File_Data"() -> (w333:refnum<vi>)
                n222 = call "DimIndicators.dic_release_service.vi"("controlRef"=w328) -> ()  [unwired: 18 in, 1 out]
                n223 = call "DimIndicators.dic_release_service.vi"("controlRef"=w329) -> ()  [unwired: 18 in, 1 out]
                n224 = call "DimIndicators.dic_release_service.vi"("controlRef"=w333) -> ()  [unwired: 18 in, 1 out]
              }
              frame #1 {
                # "Close Front Panel"
                n225 = Current VI's Path() -> (path=w348:path)
                n226 = Open VI Reference(vi path=w348) -> (vi reference=w346:refnum<vi>, error out=w345:errorcluster)  [unwired: 5 in]
                n227 = property class="VI"(reference=w346, error in=w345, "Front Panel Window:Open"=FALSE) -> ()  [unwired: 2 out]
              }
            }
            n228 = event-data() -> ()  [unwired: 2 in, 1 out]
          }
        }
      }
    }
    frame #3 {
      n229 = stacked-sequence {
        tunnel: w352 -> [w355 _ _]
        tunnel: w351 -> [w359 _ _]
        tunnel: w350 -> [w356 _ _]
        tunnel: w349 -> [w357 _ _]
        frame #0 {
          n230 = control-ref of="ListOfBases_Data"() -> (w353:refnum<vi>)
          n231 = control-ref of="Last Loaded File_Data"() -> (w358:refnum<vi>)
          n232 = control-ref of="SetFileLocation_Data"() -> (w354:refnum<vi>)
          n233 = call "DimIndicators.dic_release_service.vi"("controlRef"=w353) -> ()  [unwired: 18 in, 1 out]
          n234 = call "DimIndicators.dic_release_service.vi"("controlRef"=w358) -> ()  [unwired: 18 in, 1 out]
          n235 = call "DimIndicators.dic_release_service.vi"("controlRef"=w354) -> ()  [unwired: 18 in, 1 out]
          n236 = for "For Each Service" {
            tunnel: w357 -> [w367] mode=indexing
            n237 = Not A Number/Path/Refnum?(number/path/refnum=w367) -> (NaN/Path/Refnum?=w366:bool)
            n238 = case "Not a Reference?" shown="False" w366 {
              tunnel: w367 -> [w368 _]
              frame False {
                n239 = call "DimIndicators.dic_release_service.vi"("controlRef"=w368) -> ()  [unwired: 18 in, 1 out]
              }
              frame True {
              }
            }
          }
          n240 = for "For Each Service" {
            tunnel: w356 -> [w364] mode=indexing
            n241 = Not A Number/Path/Refnum?(number/path/refnum=w364) -> (NaN/Path/Refnum?=w363:bool)
            n242 = case "Not a Reference?" shown="False" w363 {
              tunnel: w364 -> [w365 _]
              frame False {
                n243 = call "DimIndicators.dic_release_service.vi"("controlRef"=w365) -> ()  [unwired: 18 in, 1 out]
              }
              frame True {
              }
            }
          }
          n244 = for "For Each Service" {
            tunnel: w355 -> [w361] mode=indexing
            n245 = Not A Number/Path/Refnum?(number/path/refnum=w361) -> (NaN/Path/Refnum?=w360:bool)
            n246 = case "Not a Reference?" shown="False" w360 {
              tunnel: w361 -> [w362 _]
              frame False {
                n247 = call "DimIndicators.dic_release_service.vi"("controlRef"=w362) -> ()  [unwired: 18 in, 1 out]
              }
              frame True {
              }
            }
          }
          n248 = for "Close Open Panels" {
            tunnel: w359 -> [w369] mode=indexing
            n249 = call "PanelClose.vi"("vi reference"=w369) -> ()
          }
        }
        frame #1 {
          # "Close Front Panel"
          n250 = Current VI's Path() -> (path=w373:path)
          n251 = Open VI Reference(vi path=w373) -> (vi reference=w371:refnum<vi>, error out=w370:errorcluster)  [unwired: 5 in]
          n252 = property class="VI"(reference=w371, error in=w370, "Front Panel Window:Open"=FALSE) -> ()  [unwired: 2 out]
        }
        frame #2 {
          # "Stop Panel"
          n253 = Stop(stop? (T)=TRUE) -> ()
        }
      }
    }
  }
  n254 = call "LVDimInterface.dim_operate.vi"("DNSNode"="lebit-balcony" ("DNS node")) -> ()  [unwired: 19 in]
